vi "QCA.vi"() -> ()   [LabVIEW 2009]
uses:
  QCA Global.vi
panel:
  out "Sweep Done":refnum<k4>
  out "Mode Changed":refnum<k4>
  in  "stop":bool
  in  "Mode":T1(ring)
  out "QCA Message Type":T2(ring)=enum."MonitorDelay="
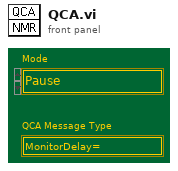
[diagram p1: front panel]
types:
  T1 = enum16{"Pause", "Take Data", "One Point", "NMR Tune", "Monitor"}
  T2 = enum16{"No Message", "Bad Message", "Init", "ChannelFile=", "RF On", "RF Off", "RFFreq=", "RFMod=", "RFPower=", "YaleGain=", "ScanSweeps=", "ScanSteps=", "ScanFreq=", "CalConst=", "MonitorDelay=", "Baseline=", "Baseline", "SaveChans", "Channel=", "Pause", "TakeData", "OnePoint", "NMRTune", "Monitor", "Address=", "Ping=", "Stop"}
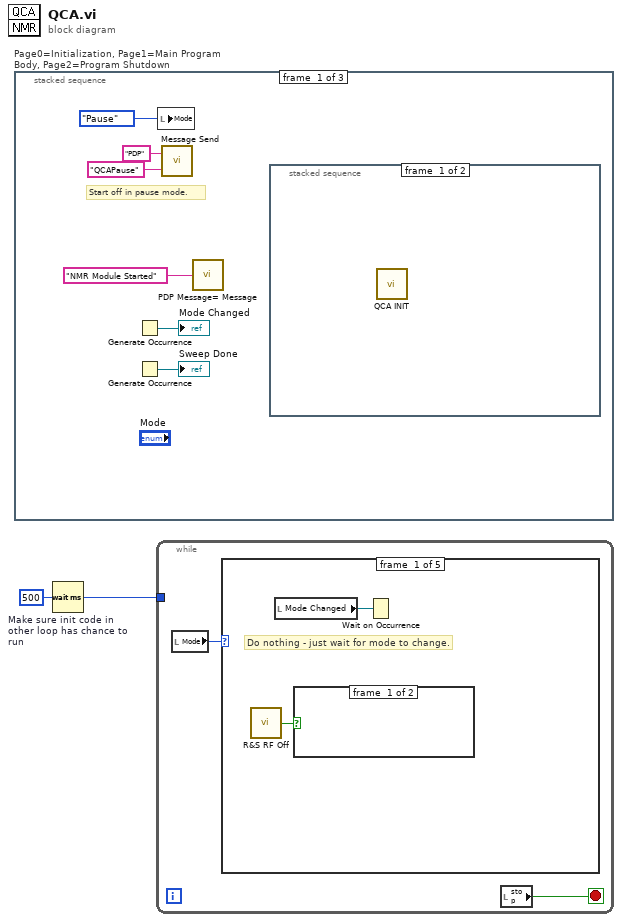
[diagram p0: block diagram]
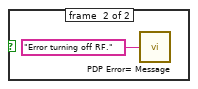
[diagram p2: hidden frame]
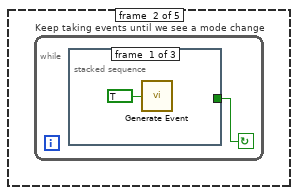
[diagram p3: hidden frame]
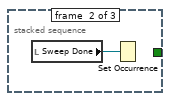
[diagram p4: hidden frame]
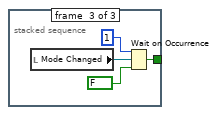
[diagram p5: hidden frame]
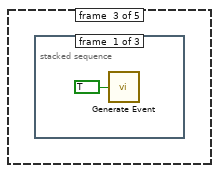
[diagram p6: hidden frame]
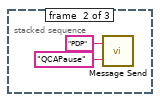
[diagram p7: hidden frame]
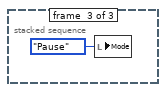
[diagram p8: hidden frame]
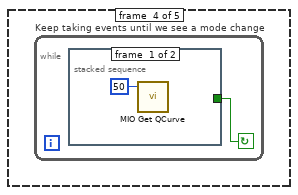
[diagram p9: hidden frame]
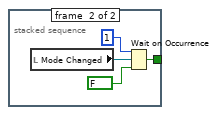
[diagram p10: hidden frame]
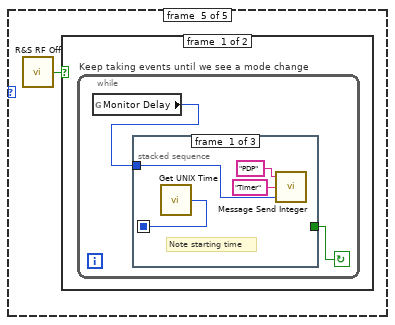
[diagram p11: hidden frame]
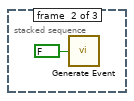
[diagram p12: hidden frame]
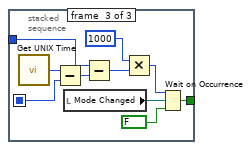
[diagram p13: hidden frame]
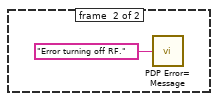
[diagram p14: hidden frame]
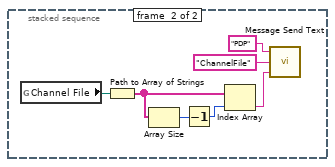
[diagram p15: hidden frame]
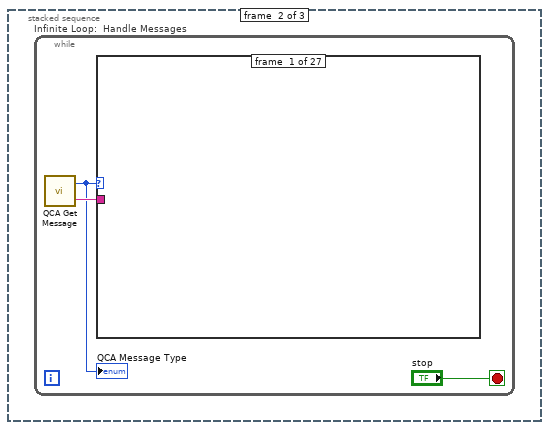
[diagram p16: hidden frame]
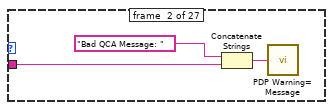
[diagram p17: hidden frame]
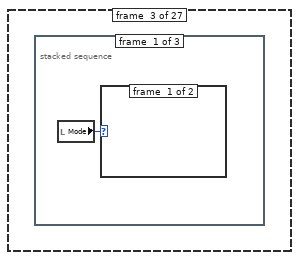
[diagram p18: hidden frame]
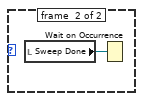
[diagram p19: hidden frame]
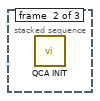
[diagram p20: hidden frame]
diagram:
  n1 = stacked-sequence "Page0=Initialization, Page1=Main Program Body, Page2=Program Shutdown" {
    frame #0 {
      # "Start off in pause mode."
      n2 = Generate Occurrence() -> (→"Mode Changed":refnum<k4>)
      n3 = Generate Occurrence() -> (→"Sweep Done":refnum<k4>)
      n4 = local write "Mode"(T1."Pause" ("Mode")) -> ()
      n5 = call "Message Send.vi"("Message"="QCAPause", "Destination"="PDP") -> ()
      n6 = call "PDP Message= Message.vi"("Message"="NMR Module Started") -> ()
      n7 = stacked-sequence {
        frame #0 {
          n8 = call "QCA INIT.vi"() -> ()  [unwired: 1 in]
        }
        frame #1 {
          n9 = global read "QCA Global.vi" "Channel File"() -> (w15:path)
          n10 = Path to Array of Strings(0:w15) -> (2:w11:string[])  [unwired: 1 out]
          n11 = Array Size(array=w11) -> (size(s)=w10:i32)
          n12 = Decrement(x=w10) -> (x-1=w9:i32)
          n13 = Index Array(array=w11, index=w9) -> (element=w12:string)
          n14 = call "Message Send Text.vi"("Value"=w12, "Parameter"="ChannelFile", "Destination"="PDP") -> ()
        }
      }
    }
    frame #1 {
      n15 = while "Infinite Loop:  Handle Messages" {
        stop <- "stop" stop-if-true
        n16 = call "QCA Get Message.vi"() -> ("QCA Message Type"=w17:T2, "Text"=w18:string)  [unwired: 1 in]
        "QCA Message Type" <- w17
        n17 = case shown="\"YaleGain=\"" w17 {
          tunnel: w18 -> [_ w19 _ w25 _ _ w40 w51 w62 w73 w86 w88 w104 w108 w110 w112 _ _ w133 _ _ _ _ _ w185 w188 _]
          frame #0 {
          }
          frame #1 {
            n18 = Concatenate Strings("Bad QCA Message: ", w19) -> (w20:string)
            n19 = call "PDP Warning= Message.vi"("Message"=w20) -> ()
          }
          frame #2 {
            n20 = stacked-sequence {
              frame #0 {
                n21 = local read "Mode"() -> (w22:T1)
                n22 = case shown="\"Take Data\"" w22 {
                  frame #0 {
                  }
                  frame #1 {
                    n23 = local read "Sweep Done"() -> (w23:refnum<k4>)
                    n24 = Wait on Occurrence(2:w23) -> ()  [unwired: 2 in, 1 out]
                  }
                }
              }
              frame #1 {
                n25 = call "QCA INIT.vi"() -> ()  [unwired: 1 in]
              }
              frame #2 {
                n26 = call "PDP Message= Message.vi"("Message"="QCA Initialized") -> ()
              }
            }
          }
          frame #3 {
            n27 = stacked-sequence {
              tunnel: w25 -> [_ w31 _ _]
              frame #0 {
                n28 = local read "Mode"() -> (w26:T1)
                n29 = case shown="\"Take Data\"" w26 {
                  frame #0 {
                  }
                  frame #1 {
                    n30 = local read "Sweep Done"() -> (w27:refnum<k4>)
                    n31 = Wait on Occurrence(2:w27) -> ()  [unwired: 2 in, 1 out]
                  }
                }
              }
              frame #1 {
                n32 = Build Array(w31) -> (w29:string[])
                n33 = Array of Strings to Path(0:w29, 1:TRUE ("relative")) -> (2:w30:path)
                n34 = global write "QCA Global.vi" "Channel File"(w30) -> ()
              }
              frame #2 {
                n35 = stacked-sequence "Read channels and set channel 0 as active." {
                  frame #0 {
                    n36 = global write "QCA Global.vi" "Current Channel"(-1 ("Current Channel")) -> ()
                  }
                  frame #1 {
                    n37 = call "QCA Init Channels.vi"() -> ()  [unwired: 1 in]
                  }
                  frame #2 {
                    n38 = call "QCA Get Channel Names.vi"() -> ("Channel Names"=w33:string[])
                    n39 = call "PDP Channels= Message.vi"("Channel"=w33) -> ()
                  }
                  frame #3 {
                    n40 = call "QCA Change Channels.vi"("Channel"=0) -> ()
                  }
                  frame #4 {
                    n41 = global read "QCA Global.vi" "Current Channel"() -> (w37:i32)
                    n42 = call "Message Send Integer.vi"("Value"=w37, "Parameter"="Channel", "Destination"="PDP") -> ()
                  }
                }
              }
              frame #3 {
                n43 = call "PDP Message= Message.vi"("Message"="Channel File Loaded") -> ()
              }
            }
          }
          frame #4 {
            n44 = call "R&S RF On.vi"() -> ()  [unwired: 1 out]
          }
          frame #5 {
            n45 = call "R&S RF Off.vi"() -> ()  [unwired: 1 out]
          }
          frame #6 {
            n46 = Fract/Exp String To Number(string=w40) -> (number=w39:dbl)  [unwired: 3 in, 1 out]
            n47 = stacked-sequence {
              tunnel: w39 -> [_ w43 w44]
              frame #0 {
                n48 = local read "Mode"() -> (w41:T1)
                n49 = case shown="\"Take Data\"" w41 {
                  frame #0 {
                  }
                  frame #1 {
                    n50 = local read "Sweep Done"() -> (w42:refnum<k4>)
                    n51 = Wait on Occurrence(2:w42) -> ()  [unwired: 2 in, 1 out]
                  }
                }
              }
              frame #1 {
                n52 = global write "QCA Global.vi" "RFFreq"(w43) -> ()
              }
              frame #2 {
                n53 = call "R&S Set RF.vi"() -> ("Error"=w45:bool)
                n54 = case shown="False" w45 {
                  tunnel: w44 -> [w46 _]
                  frame #0 {
                    n55 = call "Message Send Float.vi"("Value"=w46, "Parameter"="RFFreq", "Destination"="PDP") -> ()
                  }
                  frame #1 {
                    n56 = call "PDP Error= Message.vi"("Message"="Error=Error Setting RF Frequency.") -> ()
                  }
                }
              }
            }
          }
          frame #7 {
            n57 = Decimal String To Number(string=w51) -> (number=w50:i32)  [unwired: 2 in, 1 out]
            n58 = stacked-sequence {
              tunnel: w50 -> [_ w54 w55]
              frame #0 {
                n59 = local read "Mode"() -> (w52:T1)
                n60 = case shown="\"Take Data\"" w52 {
                  frame #0 {
                  }
                  frame #1 {
                    n61 = local read "Sweep Done"() -> (w53:refnum<k4>)
                    n62 = Wait on Occurrence(2:w53) -> ()  [unwired: 2 in, 1 out]
                  }
                }
              }
              frame #1 {
                n63 = global write "QCA Global.vi" "RFMod"(w54) -> ()
              }
              frame #2 {
                n64 = call "R&S Set RF.vi"() -> ("Error"=w56:bool)
                n65 = case shown="False" w56 {
                  tunnel: w55 -> [w59 _]
                  frame #0 {
                    n66 = call "Message Send Integer.vi"("Value"=w59, "Parameter"="RFMod", "Destination"="PDP") -> ()
                  }
                  frame #1 {
                    n67 = call "PDP Error= Message.vi"("Message"="Error=Error Setting RF Modulation.") -> ()
                  }
                }
              }
            }
          }
          frame #8 {
            n68 = Decimal String To Number(string=w62) -> (number=w61:i32)  [unwired: 2 in, 1 out]
            n69 = stacked-sequence {
              tunnel: w61 -> [_ w65 w66]
              frame #0 {
                n70 = local read "Mode"() -> (w63:T1)
                n71 = case shown="\"Take Data\"" w63 {
                  frame #0 {
                  }
                  frame #1 {
                    n72 = local read "Sweep Done"() -> (w64:refnum<k4>)
                    n73 = Wait on Occurrence(2:w64) -> ()  [unwired: 2 in, 1 out]
                  }
                }
              }
              frame #1 {
                n74 = global write "QCA Global.vi" "RFPower"(w65) -> ()
              }
              frame #2 {
                n75 = call "R&S Set RF.vi"() -> ("Error"=w67:bool)
                n76 = case shown="False" w67 {
                  tunnel: w66 -> [w70 _]
                  frame #0 {
                    n77 = call "Message Send Integer.vi"("Value"=w70, "Parameter"="RFPower", "Destination"="PDP") -> ()
                  }
                  frame #1 {
                    n78 = call "PDP Error= Message.vi"("Message"="Error=Error Setting RF Power.") -> ()
                  }
                }
              }
            }
          }
          frame #9 {
            n79 = Decimal String To Number(string=w73) -> (number=w72:i32)  [unwired: 2 in, 1 out]
            n80 = stacked-sequence {
              tunnel: w72 -> [_ w76 w77]
              frame #0 {
                n81 = local read "Mode"() -> (w74:T1)
                n82 = case shown="\"Take Data\"" w74 {
                  frame #0 {
                  }
                  frame #1 {
                    n83 = local read "Sweep Done"() -> (w75:refnum<k4>)
                    n84 = Wait on Occurrence(2:w75) -> ()  [unwired: 2 in, 1 out]
                  }
                }
              }
              frame #1 {
                n85 = global write "QCA Global.vi" "YaleGain"(w76) -> ()
              }
              frame #2 {
                n86 = call "Yale Set Gain.vi"() -> ("Error"=w78:bool)
                n87 = case shown="False" w78 {
                  tunnel: w77 -> [w81 _]
                  frame #0 {
                    n88 = call "Message Send Integer.vi"("Value"=w81, "Parameter"="YaleGain", "Destination"="PDP") -> ()
                  }
                  frame #1 {
                    n89 = call "PDP Error= Message.vi"("Message"="Error=Error Setting Yale Gain.") -> ()
                  }
                }
              }
            }
          }
          frame #10 {
            n90 = Decimal String To Number(string=w86) -> (number=w85:i32)  [unwired: 2 in, 1 out]
            n91 = global write "QCA Global.vi" "ScanSweeps"(w85) -> ()
            n92 = call "Message Send Integer.vi"("Value"=w85, "Parameter"="ScanSweeps", "Destination"="PDP") -> ()
          }
          frame #11 {
            n93 = Decimal String To Number(string=w88) -> (number=w87:i32)  [unwired: 2 in, 1 out]
            n94 = stacked-sequence {
              tunnel: w87 -> [w89 w93 w100]
              frame #0 {
                n95 = global write "QCA Global.vi" "ScanSteps"(w89) -> ()
              }
              frame #1 {
                # "setup ramp"
                n96 = for {
                  N: w93 -> [_]
                  tunnel: [w97] -> w96 mode=indexing
                  i -> [w97]
                }
                n97 = Compound Arithmetic op=MULTIPLY(w96, invert w93, 2 ("Input")) -> (w94:dbl[])
                n98 = Decrement(x=w94) -> (x-1=w91:dbl[])
                n99 = Reverse 1D Array(array=w91) -> (reversed array=w92:dbl[])
                n100 = Build Array (concatenate)(w91, w92) -> (w90:dbl[])
                n101 = global write "QCA Global.vi" "ScanRamp"(w90) -> ()
              }
              frame #2 {
                n102 = call "Message Send Integer.vi"("Value"=w100, "Parameter"="ScanSteps", "Destination"="PDP") -> ()
              }
            }
          }
          frame #12 {
            n103 = Decimal String To Number(string=w104) -> (number=w103:i32)  [unwired: 2 in, 1 out]
            n104 = global write "QCA Global.vi" "ScanFreq"(w103) -> ()
            n105 = call "Message Send Integer.vi"("Value"=w103, "Parameter"="ScanFreq", "Destination"="PDP") -> ()
          }
          frame #13 {
            n106 = Fract/Exp String To Number(string=w108) -> (number=w107:dbl)  [unwired: 3 in, 1 out]
            n107 = global write "QCA Global.vi" "CalConst"(w107) -> ()
            n108 = call "Message Send Float.vi"("Value"=w107, "Parameter"="CalConst", "Destination"="PDP") -> ()
          }
          frame #14 {
            n109 = Decimal String To Number(string=w110) -> (number=w109:i32)  [unwired: 2 in, 1 out]
            n110 = global write "QCA Global.vi" "Monitor Delay"(w109) -> ()
          }
          frame #15 {
            n111 = Decimal String To Number(string=w112) -> (number=w111:i32)  [unwired: 2 in, 1 out]
            n112 = case shown="1, Default" w111 {
              tunnel: w111 -> [_ _ w119]
              tunnel: ["New Baseline" ("TimeStamp") "No Baseline" ("TimeStamp") w118] -> w113
              frame #0 {
              }
              frame #1 {
              }
              frame #2 {
                n113 = call "Event Number to Timestamp.vi"("Event Number"=w119) -> ("TimeStamp"=w118:string)
              }
            }
            n114 = global write "QCA Global.vi" "Baseline"(w111) -> ()
            n115 = call "Message Send Text.vi"("Value"=w113, "Parameter"="Baseline", "Destination"="PDP") -> ()
          }
          frame #16 {
            n116 = global read "QCA Global.vi" "Baseline"() -> (w125:i32)
            n117 = global read "QCA Global.vi" "QMeterName"() -> (w124:string)
            n118 = call "QCA Pick Baseline.vi"("QMeter"=w124, "Current Baseline"=w125) -> ("New Baseline"=w120:i32)
            n119 = case shown="1, Default" w120 {
              tunnel: w120 -> [_ _ w129]
              tunnel: ["New Baseline" ("TimeStamp") "No Baseline" ("TimeStamp") w128] -> w121
              frame #0 {
              }
              frame #1 {
              }
              frame #2 {
                n120 = call "Event Number to Timestamp.vi"("Event Number"=w129) -> ("TimeStamp"=w128:string)
              }
            }
            n121 = global write "QCA Global.vi" "Baseline"(w120) -> ()
            n122 = call "Message Send Text.vi"("Value"=w121, "Parameter"="Baseline", "Destination"="PDP") -> ()
          }
          frame #17 {
            n123 = call "QCA Save Channels.vi"() -> ("Error"=w130:bool)
            n124 = case shown="False" w130 {
              frame #0 {
                n125 = call "PDP Message= Message.vi"("Message"="Channels Saved.") -> ()
              }
              frame #1 {
                n126 = call "PDP Error= Message.vi"("Message"="Error saving channels.") -> ()
              }
            }
          }
          frame #18 {
            n127 = stacked-sequence {
              tunnel: w133 -> [_ w137]
              frame #0 {
                n128 = local read "Mode"() -> (w134:T1)
                n129 = case shown="\"Take Data\"" w134 {
                  frame #0 {
                  }
                  frame #1 {
                    n130 = local read "Sweep Done"() -> (w135:refnum<k4>)
                    n131 = Wait on Occurrence(2:w135) -> ()  [unwired: 2 in, 1 out]
                  }
                }
              }
              frame #1 {
                n132 = Decimal String To Number(string=w137) -> (number=w136:i32)  [unwired: 2 in, 1 out]
                n133 = call "QCA Change Channels.vi"("Channel"=w136) -> ()
              }
            }
          }
          frame #19 {
            n134 = stacked-sequence {
              frame #0 {
                n135 = local read "Mode"() -> (w138:T1)
                n136 = case shown="\"Take Data\"" w138 {
                  frame #0 {
                  }
                  frame #1 {
                    n137 = local read "Sweep Done"() -> (w139:refnum<k4>)
                    n138 = Wait on Occurrence(2:w139) -> ()  [unwired: 2 in, 1 out]
                  }
                }
              }
              frame #1 {
                n139 = local write "Mode"(T1."Pause" ("Mode")) -> ()
              }
              frame #2 {
                n140 = local read "Mode Changed"() -> (w141:refnum<k4>)
                n141 = Set Occurrence(w141) -> ()
              }
              frame #3 {
                n142 = call "Message Send.vi"("Message"="QCAPause", "Destination"="PDP") -> ()
              }
            }
          }
          frame #20 {
            n143 = call "R&S RF On.vi"() -> ("Error"=w144:bool)
            n144 = case shown="False" w144 {
              frame #0 {
                n145 = stacked-sequence {
                  frame #0 {
                    n146 = local write "Mode"(T1."Take Data" ("Mode")) -> ()
                  }
                  frame #1 {
                    n147 = local read "Mode Changed"() -> (w146:refnum<k4>)
                    n148 = Set Occurrence(w146) -> ()
                  }
                  frame #2 {
                    n149 = call "Message Send.vi"("Message"="QCATakeData", "Destination"="PDP") -> ()
                  }
                }
              }
              frame #1 {
                n150 = stacked-sequence {
                  frame #0 {
                    n151 = local write "Mode"(T1."Pause" ("Mode")) -> ()
                  }
                  frame #1 {
                    n152 = local read "Mode Changed"() -> (w150:refnum<k4>)
                    n153 = Set Occurrence(w150) -> ()
                  }
                  frame #2 {
                    n154 = call "Message Send.vi"("Message"="QCAPause", "Destination"="PDP") -> ()
                  }
                  frame #3 {
                    n155 = call "PDP Error= Message.vi"("Message"="Error turning on RF.") -> ()
                  }
                }
              }
            }
          }
          frame #21 {
            n156 = call "R&S RF On.vi"() -> ("Error"=w154:bool)
            n157 = case shown="False" w154 {
              frame #0 {
                n158 = stacked-sequence {
                  frame #0 {
                    n159 = local write "Mode"(T1."One Point" ("Mode")) -> ()
                  }
                  frame #1 {
                    n160 = local read "Mode Changed"() -> (w156:refnum<k4>)
                    n161 = Set Occurrence(w156) -> ()
                  }
                  frame #2 {
                    n162 = call "Message Send.vi"("Message"="QCATakeData", "Destination"="PDP") -> ()
                  }
                }
              }
              frame #1 {
                n163 = stacked-sequence {
                  frame #0 {
                    n164 = local write "Mode"(T1."Pause" ("Mode")) -> ()
                  }
                  frame #1 {
                    n165 = local read "Mode Changed"() -> (w160:refnum<k4>)
                    n166 = Set Occurrence(w160) -> ()
                  }
                  frame #2 {
                    n167 = call "Message Send.vi"("Message"="QCAPause", "Destination"="PDP") -> ()
                  }
                  frame #3 {
                    n168 = call "PDP Error= Message.vi"("Message"="Error turning on RF.") -> ()
                  }
                }
              }
            }
          }
          frame #22 {
            n169 = stacked-sequence {
              frame #0 {
                n170 = local read "Mode"() -> (w164:T1)
                n171 = case shown="\"Take Data\"" w164 {
                  frame #0 {
                  }
                  frame #1 {
                    n172 = local read "Sweep Done"() -> (w165:refnum<k4>)
                    n173 = Wait on Occurrence(2:w165) -> ()  [unwired: 2 in, 1 out]
                  }
                }
              }
              frame #1 {
                n174 = call "R&S RF On.vi"() -> ("Error"=w166:bool)
                n175 = case shown="False" w166 {
                  frame #0 {
                    n176 = stacked-sequence {
                      frame #0 {
                        n177 = local write "Mode"(T1."NMR Tune" ("Mode")) -> ()
                      }
                      frame #1 {
                        n178 = local read "Mode Changed"() -> (w168:refnum<k4>)
                        n179 = Set Occurrence(w168) -> ()
                      }
                      frame #2 {
                        n180 = call "Message Send.vi"("Message"="QCANMRTune", "Destination"="PDP") -> ()
                      }
                    }
                  }
                  frame #1 {
                    n181 = stacked-sequence {
                      frame #0 {
                        n182 = local write "Mode"(T1."Pause" ("Mode")) -> ()
                      }
                      frame #1 {
                        n183 = local read "Mode Changed"() -> (w172:refnum<k4>)
                        n184 = Set Occurrence(w172) -> ()
                      }
                      frame #2 {
                        n185 = call "Message Send.vi"("Message"="QCAPause", "Destination"="PDP") -> ()
                      }
                      frame #3 {
                        n186 = call "PDP Error= Message.vi"("Message"="Error turning on RF.") -> ()
                      }
                    }
                  }
                }
              }
            }
          }
          frame #23 {
            n187 = stacked-sequence {
              frame #0 {
                n188 = local read "Mode"() -> (w176:T1)
                n189 = case shown="\"Take Data\"" w176 {
                  frame #0 {
                  }
                  frame #1 {
                    n190 = local read "Sweep Done"() -> (w177:refnum<k4>)
                    n191 = Wait on Occurrence(2:w177) -> ()  [unwired: 2 in, 1 out]
                  }
                }
              }
              frame #1 {
                n192 = local write "Mode"(T1."Monitor" ("Mode")) -> ()
              }
              frame #2 {
                n193 = local read "Mode Changed"() -> (w179:refnum<k4>)
                n194 = Set Occurrence(w179) -> ()
              }
              frame #3 {
                n195 = call "Message Send.vi"("Message"="QCAMonitor", "Destination"="PDP") -> ()
              }
            }
          }
          frame #24 {
            n196 = Scan From String(format string="%s,%[.0-9]:%d" ("Format String"), input string=w185) -> (output 1=w183:string, output 2=w184:string, output 3=w182:i32)  [unwired: 5 in, 3 out]
            n197 = call "Message Set Module Address.vi"("Port"=w182, "Address"=w184, "Module"=w183) -> ()
          }
          frame #25 {
            n198 = Get Date/Time In Seconds() -> (seconds since 1Jan1904=w187:timestamp)
            n199 = To Double Precision Float(number=w187) -> (double precision float=w190:dbl)
            n200 = Format Into String(format string="PingResponse=QCA,%.0f", w190) -> (resulting string=w189:string)  [unwired: 2 in, 1 out]
            n201 = call "Message Send.vi"("Message"=w189, "Destination"=w188) -> ()
          }
          frame #26 {
            n202 = local write "stop"(TRUE ("stop")) -> ()
          }
        }
      }
    }
    frame #2 {
      n203 = call "PDP Message= Message.vi"("Message"="QCA Module Stopped") -> ()
    }
  }
  n204 = Wait (ms) "Make sure init code in other loop has chance to run"(milliseconds to wait=u32 500) -> (millisecond timer value=w1:u32)
  n205 = while {
    tunnel: w1 -> [_]
    stop <- w194 stop-if-true
    n206 = local read "Mode"() -> (w195:T1)
    n207 = case shown="\"Take Data\"" w195 {
      frame #0 {
        # "Do nothing - just wait for mode to change."
        n208 = call "R&S RF Off.vi"() -> ("Error"=w196:bool)
        n209 = local read "Mode Changed"() -> (w197:refnum<k4>)
        n210 = case shown="True" w196 {
          frame #0 {
          }
          frame #1 {
            n211 = call "PDP Error= Message.vi"("Message"="Error turning off RF.") -> ()
          }
        }
        n212 = Wait on Occurrence(2:w197) -> ()  [unwired: 2 in, 1 out]
      }
      frame #1 {
        n213 = while "Keep taking events until we see a mode change" {
          stop <- w199 continue-if-true
          n214 = stacked-sequence {
            tunnel: [_ _ w205] -> w199
            frame #0 {
              n215 = call "Generate Event.vi"("Include NMR Data"=TRUE) -> ()
            }
            frame #1 {
              n216 = local read "Sweep Done"() -> (w201:refnum<k4>)
              n217 = Set Occurrence(w201) -> ()
            }
            frame #2 {
              n218 = local read "Mode Changed"() -> (w204:refnum<k4>)
              n219 = Wait on Occurrence(1:FALSE ("ignore previous (T)"), 2:w204, 3:1 ("ms timeout (-1)")) -> (0:w205:bool)
            }
          }
        }
      }
      frame #2 {
        n220 = stacked-sequence {
          frame #0 {
            n221 = call "Generate Event.vi"("Include NMR Data"=TRUE) -> ()
          }
          frame #1 {
            n222 = call "Message Send.vi"("Message"="QCAPause", "Destination"="PDP") -> ()
          }
          frame #2 {
            n223 = local write "Mode"(T1."Pause" ("Mode")) -> ()
          }
        }
      }
      frame #3 {
        n224 = while "Keep taking events until we see a mode change" {
          stop <- w210 continue-if-true
          n225 = stacked-sequence {
            tunnel: [_ w215] -> w210
            frame #0 {
              n226 = call "MIO Get QCurve.vi"("Num Sweeps"=50) -> ()  [unwired: 2 in, 1 out]
            }
            frame #1 {
              n227 = local read "Mode Changed"() -> (w214:refnum<k4>)
              n228 = Wait on Occurrence(1:FALSE ("ignore previous (T)"), 2:w214, 3:1 ("ms timeout (-1)")) -> (0:w215:bool)
            }
          }
        }
      }
      frame #4 {
        n229 = call "R&S RF Off.vi"() -> ("Error"=w216:bool)
        n230 = case shown="False" w216 {
          frame #0 {
            n231 = while "Keep taking events until we see a mode change" {
              stop <- w218 continue-if-true
              n232 = global read "QCA Global.vi" "Monitor Delay"() -> (w217:i32)
              n233 = stacked-sequence {
                seq-local: [w222 _ _] -> [_ _ w231]
                tunnel: [_ _ w233] -> w218
                tunnel: w217 -> [w219 _ w225]
                frame #0 {
                  # "Note starting time"
                  n234 = call "Get UNIX Time.vi"() -> ("UNIX seconds"=w222:i32)
                  n235 = call "Message Send Integer.vi"("Value"=w219, "Parameter"="Timer", "Destination"="PDP") -> ()
                }
                frame #1 {
                  n236 = call "Generate Event.vi"("Include NMR Data"=FALSE) -> ()
                }
                frame #2 {
                  n237 = call "Get UNIX Time.vi"() -> ("UNIX seconds"=w230:i32)
                  n238 = Subtract(x=w230, y=w231) -> (x-y=w229:i32)
                  n239 = local read "Mode Changed"() -> (w232:refnum<k4>)
                  n240 = Subtract(x=w225, y=w229) -> (x-y=w228:i32)
                  n241 = Multiply(x=1000, y=w228) -> (x*y=w226:i32)
                  n242 = Wait on Occurrence(1:FALSE ("ignore previous (T)"), 2:w232, 3:w226) -> (0:w233:bool)
                }
              }
            }
          }
          frame #1 {
            n243 = call "PDP Error= Message.vi"("Message"="Error turning off RF.") -> ()
          }
        }
      }
    }
    n244 = local read "stop"() -> (w194:bool)
  }
